vi "3.feladat.vi"() -> ()   [LabVIEW 2015]
panel:
  out "Boolean 2":bool
  out "kocka2":dbl
  out "kocka1":dbl
  in  "Boolean":bool
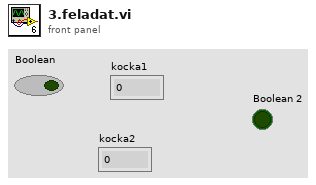
[diagram p1: front panel]
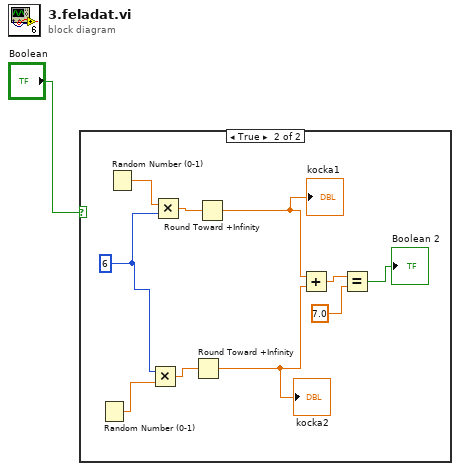
[diagram p0: block diagram]
diagram:
  n1 = case shown="True" "Boolean" {
    frame False {
    }
    frame True {
      w6 = 6
      n2 = Random Number (0-1)() -> (number: 0 to 1=w11:dbl)
      n3 = Random Number (0-1)() -> (number: 0 to 1=w10:dbl)
      n4 = Multiply(x=w6, y=w11) -> (x*y=w4:dbl)
      n5 = Multiply(x=w10, y=w6) -> (x*y=w5:dbl)
      n6 = Round Toward +Infinity(x=w4) -> (ceil(x): smallest int >= x=w2:dbl)
      "kocka2" <- w2
      n7 = Round Toward +Infinity(x=w5) -> (ceil(x): smallest int >= x=w3:dbl)
      "kocka1" <- w3
      n8 = Add(x=w3, y=w2) -> (x+y=w9:dbl)
      n9 = Equal?(x=w9, y=7.0) -> (x = y?=→"Boolean 2":bool)
    }
  }
